vi "PH_Beckhoff.set i Attr and open Services.vi"(0 "i ref in":refnum<vi>, 2 "data in":string, 5 "error in":errorcluster) -> (14 "i ref out":refnum<vi>, 16 "i Attr":T1={"GUI Refs"={"ADS Error"=refnum, "Values"=refnum, "configured?"=refnum, "Connection"=refnum, "IP"=refnum, "Prdc Int [ms]"=refnum}, "operation?"=FALSE, "Default Prdc Interval"=0, "Connection"={"DLL?"=FALSE, "Port?"=FALSE, "Client?"=FALSE, "Ping?"=FALSE, "unsuccessful Pings"=0}, "AMS Net ID"={"DLL path"=path "", "AMS Net ID"={"1st # of IP"=0, "2nd # of IP"=0, "3rd # of IP"=0, "4th # of IP"=0, "In Port"=0, "Out Port"=0}}, "Klemmencluster: # of"={"Offset due to Sonderklemms"=0, "analog Inputs"=0, "analog Outputs"=0, "digital Input Bits"=0, "digital Output Bits"=0}, "Values"={"Sonderklemmen Inputs"=[], "Analog Inputs"=[], "Analog Outputs"=[], "Digital Inputs"=[], "Digital Outputs"=[]}, "IP"="", "Description"="", "configured?"=FALSE, "Change Manager"={"Detemination wanted?"=FALSE, "Values changed at"={"Sonderklemmen Inputs"=[], "Analog Inputs"=[], "Analog Outputs"=[], "Digital Inputs"=[], "Digital Outputs"=[]}}, "Difference to handle an analog input as change"=1}, 19 "error out":errorcluster)   [LabVIEW 2014, in "PH_Beckhoff.lvlib"]
doc: "This VI opens all DIM services."
uses:
  PH_Beckhoff.lvlib
  PH_Beckhoff.i attribute.ctl
  PH_Beckhoff.GUI Refs.ctl
  PH_Beckhoff.Values.ctl
  PH_Beckhoff.Sonderklemmen Inputs.ctl
  PH_Beckhoff.Analog Inputs.ctl
  PH_Beckhoff.Scaling Type.ctl
  PH_Beckhoff.Analog Outputs.ctl
  PH_Beckhoff.Digital Inputs.ctl
  PH_Beckhoff.Digital Outputs.ctl
  PH_Beckhoff.Connectivity.ctl
  non_GPL/instr.lib/Beckhoff/Helpers/Beckhoff Access.ctl
  non_GPL/instr.lib/Beckhoff/Helpers/Klemmendeclarer.ctl
  PH_Beckhoff.constructor Data in.ctl
  lib.lib/DimLVEvent/LVDimInterface/LVDimInterface.lvlib
  non_GPL/instr.lib/Beckhoff/Beckhoff - Driver np.lvlib
  CSCore/CSSystem/CSSystemLib/CSSystemLib.lvlib
  CSCore/BaseProcess/BaseProcess.lvlib
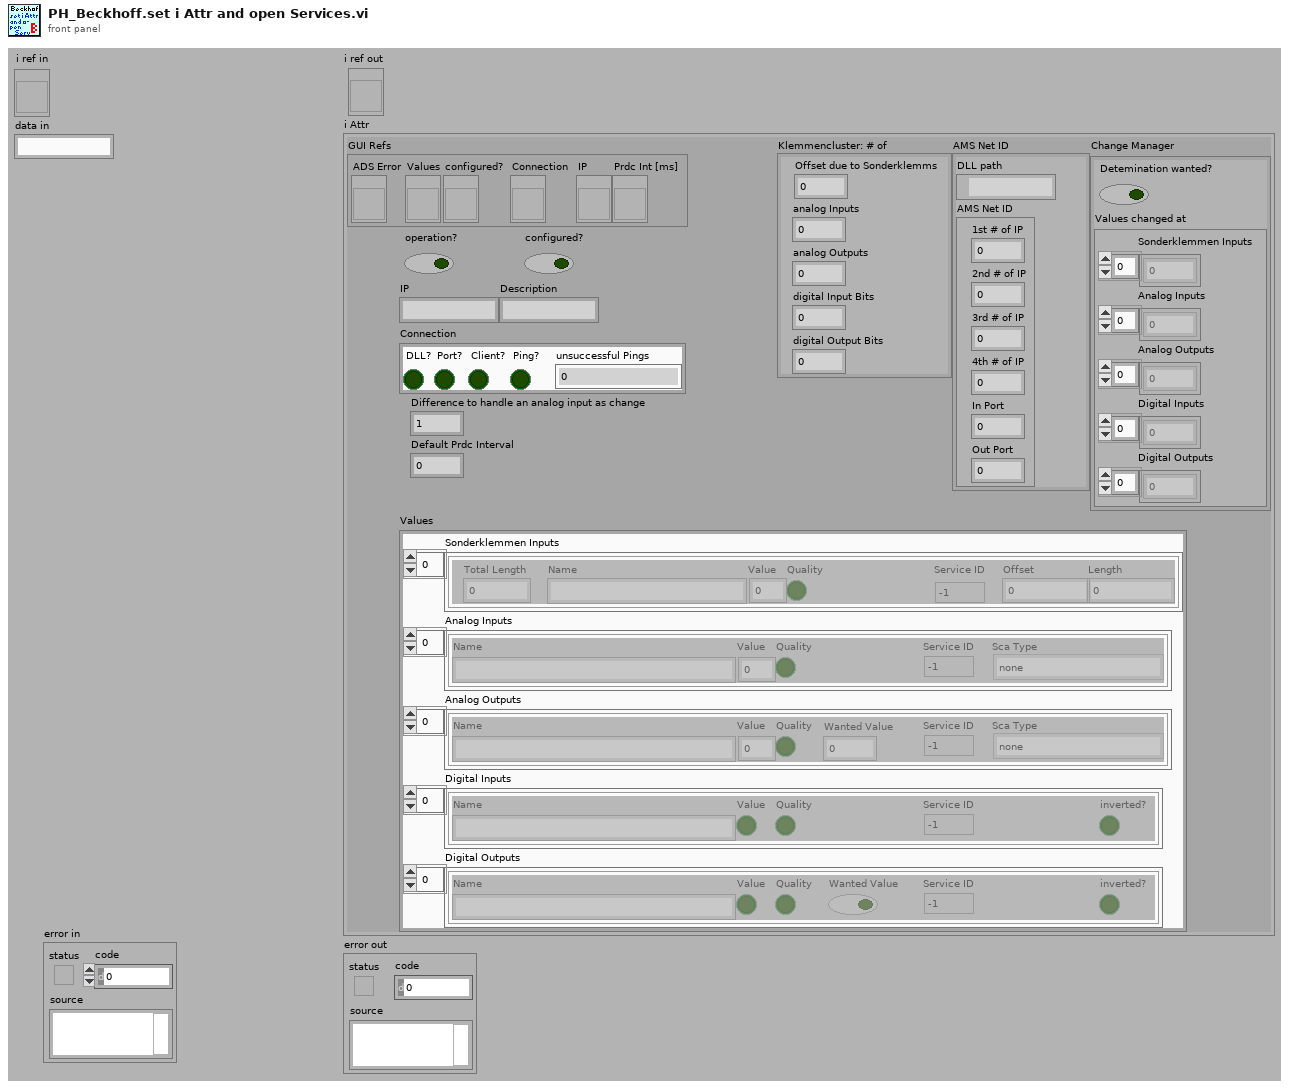
[diagram p1: front panel]
types:
  T1 = typedef "PH_Beckhoff.lvlib/PH_Beckhoff.i attribute.ctl" = cluster{"GUI Refs":T2, "operation?":bool, "Default Prdc Interval":i32, "Connection":T3, "AMS Net ID":T4, "Klemmencluster: # of":T5, "Values":T6, "IP":string, "Description":string, "configured?":bool, "Change Manager":cluster{"Detemination wanted?":bool, "Values changed at":cluster{"Sonderklemmen Inputs":i32[], "Analog Inputs":i32[], "Analog Outputs":i32[], "Digital Inputs":i32[], "Digital Outputs":i32[]}}, "Difference to handle an analog input as change":u32}
  T2 = typedef "PH_Beckhoff.lvlib/PH_Beckhoff.GUI Refs.ctl" = cluster{"ADS Error":refnum<vi>, "Values":refnum<vi>, "configured?":refnum<vi>, "Connection":refnum<vi>, "IP":refnum<vi>, "Prdc Int [ms]":refnum<vi>}
  T3 = typedef "PH_Beckhoff.lvlib/PH_Beckhoff.Connectivity.ctl" = cluster{"DLL?":bool, "Port?":bool, "Client?":bool, "Ping?":bool, "unsuccessful Pings":u32}
  T4 = typedef "Beckhoff - Driver np.lvlib/Beckhoff Access.ctl" = cluster{"DLL path":path, "AMS Net ID":cluster{"1st # of IP":u8, "2nd # of IP":u8, "3rd # of IP":u8, "4th # of IP":u8, "In Port":u8, "Out Port":u8}}
  T5 = typedef "Beckhoff - Driver np.lvlib/Klemmendeclarer.ctl" = cluster{"Offset due to Sonderklemms":u32, "analog Inputs":u32, "analog Outputs":u32, "digital Input Bits":u32, "digital Output Bits":u32}
  T6 = typedef "PH_Beckhoff.lvlib/PH_Beckhoff.Values.ctl" = cluster{"Sonderklemmen Inputs":T7, "Analog Inputs":T8, "Analog Outputs":T10, "Digital Inputs":T11, "Digital Outputs":T12}
  T7 = typedef "PH_Beckhoff.lvlib/PH_Beckhoff.Sonderklemmen Inputs.ctl" = cluster{"Total Length":u32, "Name":string, "Value":u64, "Quality":bool, "Service ID":i32, "Offset":u32, "Length":u32}[]
  T8 = typedef "PH_Beckhoff.lvlib/PH_Beckhoff.Analog Inputs.ctl" = cluster{"Name":string, "Value":u32, "Quality":bool, "Service ID":i32, "Sca Type":T9}[]
  T9 = typedef "PH_Beckhoff.lvlib/PH_Beckhoff.Scaling Type.ctl" = enum16{"none", "0 ... 15 Bit -> 0 ... 5", "0 ... 15 Bit -> 0 ... 10", "0 ... 15 Bit -> 0 ... 25", "0 ... 15 Bit -> 4 ... 20", "0 ... 15 Bit -> 0 ... 1", "0 ... 15 Bit -> 0 ... 20000", "0 ... 15 Bit -> 0 ... 24000"}
  T10 = typedef "PH_Beckhoff.lvlib/PH_Beckhoff.Analog Outputs.ctl" = cluster{"Name":string, "Value":u32, "Quality":bool, "Wanted Value":u32, "Service ID":i32, "Sca Type":T9}[]
  T11 = typedef "PH_Beckhoff.lvlib/PH_Beckhoff.Digital Inputs.ctl" = cluster{"Name":string, "Value":bool, "Quality":bool, "Service ID":i32, "inverted?":bool}[]
  T12 = typedef "PH_Beckhoff.lvlib/PH_Beckhoff.Digital Outputs.ctl" = cluster{"Name":string, "Value":bool, "Quality":bool, "Wanted Value":bool, "Service ID":i32, "inverted?":bool}[]
  T13 = typedef "PH_Beckhoff.lvlib/PH_Beckhoff.constructor Data in.ctl" = cluster{"Default Values":T6, "Description":string, "Hardware configured?":bool, "Activate Change Manager?":bool, "Difference to handle an analog input as change":u32}
  T14 = cluster{"Total Length":u32, "Name":string, "Value":u64, "Quality":bool, "Service ID":i32, "Offset":u32, "Length":u32}
  T15 = cluster{"Name":string, "Value":bool, "Quality":bool, "Wanted Value":bool, "Service ID":i32, "inverted?":bool}
  T16 = cluster{"Name":string, "Value":bool, "Quality":bool, "Service ID":i32, "inverted?":bool}
  T17 = cluster{"Name":string, "Value":u32, "Quality":bool, "Wanted Value":u32, "Service ID":i32, "Sca Type":T9}
  T18 = cluster{"Name":string, "Value":u32, "Quality":bool, "Service ID":i32, "Sca Type":T9}
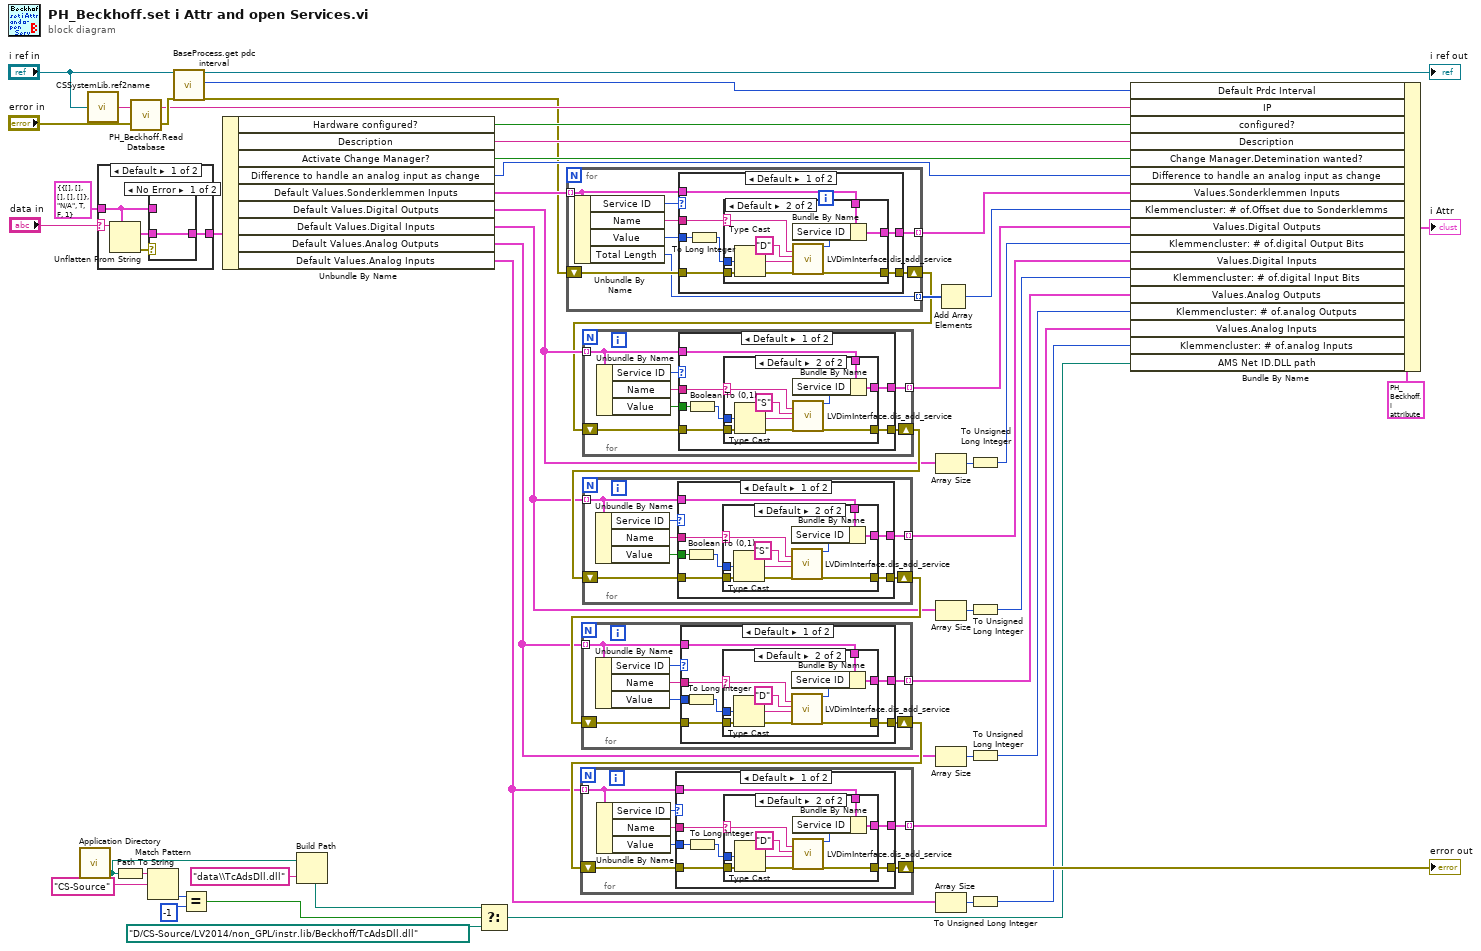
[diagram p0: block diagram]
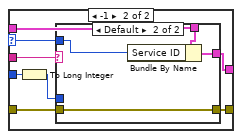
[diagram p5: hidden frame]
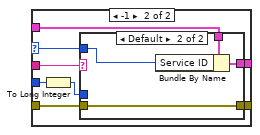
[diagram p8: hidden frame]
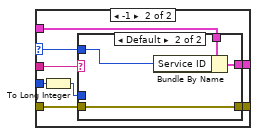
[diagram p11: hidden frame]
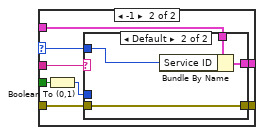
[diagram p14: hidden frame]
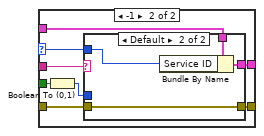
[diagram p17: hidden frame]
diagram:
  n1 = call <vilib>:"Application Directory.vi"() -> ("Application Directory"=w37:path)
  n2 = call "CSSystemLib.ref2name.vi"("obj refnum"="i ref in") -> ("name"=w1:string)
  n3 = case shown="Default" "data in" {
    selector: "data in" -> [w57 _]
    tunnel: T13 {"Default Values"={"Sonderklemmen Inputs"=[], "Analog Inputs"=[], "Analog Outputs"=[], "Digital Inputs"=[], "Digital Outputs"=[]}, "Description"="N/A", "Hardware configured?"=TRUE, "Activate Change Manager?"=FALSE, "Difference to handle an analog input as change"=1} ("data in cluster") -> [w53 w60]
    tunnel: [w54 w60] -> w31
    frame Default {
      n4 = Unflatten From String(type=w53, binary string=w57) -> (value=w55:T13, error out=w56:errorcluster)  [unwired: 3 in, 1 out]
      n5 = case shown="No Error" w56 {
        tunnel: w55 -> [w58 _]
        tunnel: [w58 w59] -> w54
        tunnel: w53 -> [_ w59]
        frame No Error {
        }
        frame Error {
        }
      }
    }
    frame "", "N/A" {
    }
  }
  n6 = Path To String(path=w37) -> (string=w32:string)
  n7 = call "PH_Beckhoff.Read Database.vi"("error in (no error)"="error in", "DB Entry to read"=w1) -> ("error out"=w10:errorcluster, "IP"=w7:string)
  n8 = Match Pattern(string=w32, regular expression="CS-Source") -> (offset past match=w34:i32)  [unwired: 1 in, 3 out]
  n9 = call "BaseProcess.get pdc interval.vi"("i ref in"="i ref in", "error in (no error)"=w10) -> ("i ref out"=→"i ref out":refnum<vi>, "PeriodicInterval"=w9:i32, "error out"=w4:errorcluster)  [unwired: 15 in]
  n10 = Equal?(x=w34, y=-1) -> (x = y?=w36:bool)
  n11 = Unbundle By Name(w31) -> ("Hardware configured?"=w8:bool, "Description"=w14:string, "Activate Change Manager?"=w13:bool, "Difference to handle an analog input as change"=w6:u32, "Default Values.Sonderklemmen Inputs"=w28:T7, "Default Values.Digital Outputs"=w27:T12, "Default Values.Digital Inputs"=w26:T11, "Default Values.Analog Outputs"=w25:T10, "Default Values.Analog Inputs"=w11:T8)
  n12 = Build Path(base path=w37, name or relative path="data\\TcAdsDll.dll") -> (appended path=w39:path)
  n13 = Select(t=w39, s=w36, f=path "D:/CS-Source/LV2014/non_GPL/instr.lib/Beckhoff/TcAdsDll.dll") -> (s? t:f=w15:path)
  n14 = for {
    shift-right: [w67] -> w21
    shift-left: w4 -> [w68]
    tunnel: [w66] -> w23 mode=indexing
    tunnel: w28 -> [w65] mode=indexing
    tunnel: [w62] -> w42 mode=indexing
    n15 = Unbundle By Name(w65) -> ("Service ID"=w61:i32, "Name"=w64:string, "Value"=w63:u64, "Total Length"=w62:u32)
    n16 = case shown="Default" w61 {
      selector: w61 -> [_ w87]
      tunnel: w68 -> [w75 w94]
      tunnel: [w74 w93] -> w67
      tunnel: [w73 w92] -> w66
      tunnel: w65 -> [w72 w91]
      tunnel: w64 -> [w71 w90]
      tunnel: w63 -> [w70 w89]
      frame Default {
        n17 = To Long Integer(number=w70) -> (32bit integer=w69:i32)
        n18 = case shown="Default" w71 {
          selector: w71 -> [_ w78]
          tunnel: w75 -> [w76 w84]
          tunnel: [w76 w83] -> w74
          tunnel: [w77 w81] -> w73
          tunnel: w72 -> [w77 w80]
          tunnel: w69 -> [_ w79]
          frame "", "N/A" {
          }
          frame Default {
            n19 = Type Cast(x=w79) -> (*(type *) &x=w86:string)  [unwired: 1 in]
            n20 = call "LVDimInterface.dis_add_service.vi"("serviceName"=w78, "typeDescriptor"="D", "data"=w86, "error in (no error)"=w84) -> ("my_serviceID"=w82:i32, "error out"=w83:errorcluster)  [unwired: 14 in]
            n21 = Bundle By Name(cluster=w80, "Service ID"=w82) -> (w81:T14)
          }
        }
      }
      frame -1 {
        n22 = To Long Integer(number=w89) -> (32bit integer=w88:i32)
        n23 = case shown="Default" w90 {
          tunnel: w94 -> [w95 w98]
          tunnel: [w95 w98] -> w93
          tunnel: [w96 w100] -> w92
          tunnel: w91 -> [w96 w99]
          tunnel: w88 -> [_ _]
          tunnel: w87 -> [_ w97]
          frame "", "N/A" {
          }
          frame Default {
            n24 = Bundle By Name(cluster=w99, "Service ID"=w97) -> (w100:T14)
          }
        }
      }
    }
  }
  n25 = for {
    shift-right: [w106] -> w45
    shift-left: w21 -> [w107]
    tunnel: [w105] -> w52 mode=indexing
    tunnel: w27 -> [w104] mode=indexing
    n26 = Unbundle By Name(w104) -> ("Service ID"=w101:i32, "Name"=w103:string, "Value"=w102:bool)
    n27 = case shown="Default" w101 {
      selector: w101 -> [_ w126]
      tunnel: w107 -> [w114 w133]
      tunnel: [w113 w132] -> w106
      tunnel: [w112 w131] -> w105
      tunnel: w104 -> [w111 w130]
      tunnel: w103 -> [w110 w129]
      tunnel: w102 -> [w109 w128]
      frame Default {
        n28 = Boolean To (0,1)(Boolean=w109) -> (0, 1=w108:i16)
        n29 = case shown="Default" w110 {
          selector: w110 -> [_ w117]
          tunnel: w114 -> [w115 w123]
          tunnel: [w115 w122] -> w113
          tunnel: [w116 w120] -> w112
          tunnel: w111 -> [w116 w119]
          tunnel: w108 -> [_ w118]
          frame "", "N/A" {
          }
          frame Default {
            n30 = Type Cast(x=w118) -> (*(type *) &x=w125:string)  [unwired: 1 in]
            n31 = call "LVDimInterface.dis_add_service.vi"("serviceName"=w117, "typeDescriptor"="S", "data"=w125, "error in (no error)"=w123) -> ("my_serviceID"=w121:i32, "error out"=w122:errorcluster)  [unwired: 14 in]
            n32 = Bundle By Name(cluster=w119, "Service ID"=w121) -> (w120:T15)
          }
        }
      }
      frame -1 {
        n33 = Boolean To (0,1)(Boolean=w128) -> (0, 1=w127:i16)
        n34 = case shown="Default" w129 {
          tunnel: w133 -> [w134 w137]
          tunnel: [w134 w137] -> w132
          tunnel: [w135 w139] -> w131
          tunnel: w130 -> [w135 w138]
          tunnel: w127 -> [_ _]
          tunnel: w126 -> [_ w136]
          frame "", "N/A" {
          }
          frame Default {
            n35 = Bundle By Name(cluster=w138, "Service ID"=w136) -> (w139:T15)
          }
        }
      }
    }
  }
  n36 = for {
    shift-right: [w145] -> w43
    shift-left: w45 -> [w146]
    tunnel: [w144] -> w51 mode=indexing
    tunnel: w26 -> [w141] mode=indexing
    n37 = Unbundle By Name(w141) -> ("Service ID"=w140:i32, "Name"=w143:string, "Value"=w142:bool)
    n38 = case shown="Default" w140 {
      selector: w140 -> [_ w165]
      tunnel: w146 -> [w153 w172]
      tunnel: [w152 w171] -> w145
      tunnel: [w151 w170] -> w144
      tunnel: w143 -> [w150 w169]
      tunnel: w142 -> [w149 w168]
      tunnel: w141 -> [w147 w166]
      frame Default {
        n39 = Boolean To (0,1)(Boolean=w149) -> (0, 1=w148:i16)
        n40 = case shown="Default" w150 {
          selector: w150 -> [_ w156]
          tunnel: w153 -> [w154 w162]
          tunnel: [w154 w161] -> w152
          tunnel: [w155 w159] -> w151
          tunnel: w147 -> [w155 w158]
          tunnel: w148 -> [_ w157]
          frame "", "N/A" {
          }
          frame Default {
            n41 = Type Cast(x=w157) -> (*(type *) &x=w164:string)  [unwired: 1 in]
            n42 = call "LVDimInterface.dis_add_service.vi"("serviceName"=w156, "typeDescriptor"="S", "data"=w164, "error in (no error)"=w162) -> ("my_serviceID"=w160:i32, "error out"=w161:errorcluster)  [unwired: 14 in]
            n43 = Bundle By Name(cluster=w158, "Service ID"=w160) -> (w159:T16)
          }
        }
      }
      frame -1 {
        n44 = Boolean To (0,1)(Boolean=w168) -> (0, 1=w167:i16)
        n45 = case shown="Default" w169 {
          tunnel: w172 -> [w173 w176]
          tunnel: [w173 w176] -> w171
          tunnel: [w174 w178] -> w170
          tunnel: w166 -> [w174 w177]
          tunnel: w167 -> [_ _]
          tunnel: w165 -> [_ w175]
          frame "", "N/A" {
          }
          frame Default {
            n46 = Bundle By Name(cluster=w177, "Service ID"=w175) -> (w178:T16)
          }
        }
      }
    }
  }
  n47 = for {
    shift-right: [w184] -> w44
    shift-left: w43 -> [w185]
    tunnel: [w183] -> w50 mode=indexing
    tunnel: w25 -> [w182] mode=indexing
    n48 = Unbundle By Name(w182) -> ("Service ID"=w179:i32, "Name"=w181:string, "Value"=w180:u32)
    n49 = case shown="Default" w179 {
      selector: w179 -> [_ w204]
      tunnel: w185 -> [w192 w211]
      tunnel: [w191 w210] -> w184
      tunnel: [w190 w209] -> w183
      tunnel: w182 -> [w189 w208]
      tunnel: w181 -> [w188 w207]
      tunnel: w180 -> [w187 w206]
      frame Default {
        n50 = To Long Integer(number=w187) -> (32bit integer=w186:i32)
        n51 = case shown="Default" w188 {
          selector: w188 -> [_ w195]
          tunnel: w192 -> [w193 w201]
          tunnel: [w193 w200] -> w191
          tunnel: [w194 w198] -> w190
          tunnel: w189 -> [w194 w197]
          tunnel: w186 -> [_ w196]
          frame "", "N/A" {
          }
          frame Default {
            n52 = Type Cast(x=w196) -> (*(type *) &x=w203:string)  [unwired: 1 in]
            n53 = call "LVDimInterface.dis_add_service.vi"("serviceName"=w195, "typeDescriptor"="D", "data"=w203, "error in (no error)"=w201) -> ("my_serviceID"=w199:i32, "error out"=w200:errorcluster)  [unwired: 14 in]
            n54 = Bundle By Name(cluster=w197, "Service ID"=w199) -> (w198:T17)
          }
        }
      }
      frame -1 {
        n55 = To Long Integer(number=w206) -> (32bit integer=w205:i32)
        n56 = case shown="Default" w207 {
          tunnel: w211 -> [w212 w215]
          tunnel: [w212 w215] -> w210
          tunnel: [w213 w217] -> w209
          tunnel: w208 -> [w213 w216]
          tunnel: w205 -> [_ _]
          tunnel: w204 -> [_ w214]
          frame "", "N/A" {
          }
          frame Default {
            n57 = Bundle By Name(cluster=w216, "Service ID"=w214) -> (w217:T17)
          }
        }
      }
    }
  }
  n58 = for {
    shift-right: [w223] -> w20
    shift-left: w44 -> [w224]
    tunnel: [w222] -> w12 mode=indexing
    tunnel: w11 -> [w221] mode=indexing
    n59 = Unbundle By Name(w221) -> ("Service ID"=w218:i32, "Name"=w220:string, "Value"=w219:u32)
    n60 = case shown="Default" w218 {
      selector: w218 -> [_ w243]
      tunnel: w224 -> [w231 w250]
      tunnel: [w230 w249] -> w223
      tunnel: [w229 w248] -> w222
      tunnel: w221 -> [w228 w247]
      tunnel: w220 -> [w227 w246]
      tunnel: w219 -> [w226 w245]
      frame Default {
        n61 = To Long Integer(number=w226) -> (32bit integer=w225:i32)
        n62 = case shown="Default" w227 {
          selector: w227 -> [_ w234]
          tunnel: w231 -> [w232 w240]
          tunnel: [w232 w239] -> w230
          tunnel: [w233 w237] -> w229
          tunnel: w228 -> [w233 w236]
          tunnel: w225 -> [_ w235]
          frame "", "N/A" {
          }
          frame Default {
            n63 = Type Cast(x=w235) -> (*(type *) &x=w242:string)  [unwired: 1 in]
            n64 = call "LVDimInterface.dis_add_service.vi"("serviceName"=w234, "typeDescriptor"="D", "data"=w242, "error in (no error)"=w240) -> ("my_serviceID"=w238:i32, "error out"=w239:errorcluster)  [unwired: 14 in]
            n65 = Bundle By Name(cluster=w236, "Service ID"=w238) -> (w237:T18)
          }
        }
      }
      frame -1 {
        n66 = To Long Integer(number=w245) -> (32bit integer=w244:i32)
        n67 = case shown="Default" w246 {
          tunnel: w250 -> [w251 w254]
          tunnel: [w251 w254] -> w249
          tunnel: [w252 w256] -> w248
          tunnel: w247 -> [w252 w255]
          tunnel: w244 -> [_ _]
          tunnel: w243 -> [_ w253]
          frame "", "N/A" {
          }
          frame Default {
            n68 = Bundle By Name(cluster=w255, "Service ID"=w253) -> (w256:T18)
          }
        }
      }
    }
  }
  "error out" <- w20
  n69 = Array Size(array=w27) -> (size(s)=w49:i32)
  n70 = Array Size(array=w26) -> (size(s)=w46:i32)
  n71 = Array Size(array=w25) -> (size(s)=w47:i32)
  n72 = Array Size(array=w11) -> (size(s)=w48:i32)
  n73 = Add Array Elements(numeric array=w42) -> (sum=w22:u32)
  n74 = To Unsigned Long Integer(number=w49) -> (unsigned 32bit integer=w19:u32)
  n75 = To Unsigned Long Integer(number=w46) -> (unsigned 32bit integer=w18:u32)
  n76 = To Unsigned Long Integer(number=w47) -> (unsigned 32bit integer=w17:u32)
  n77 = To Unsigned Long Integer(number=w48) -> (unsigned 32bit integer=w16:u32)
  n78 = Bundle By Name(cluster=T1 {"GUI Refs"={"ADS Error"=refnum, "Values"=refnum, "configured?"=refnum, "Connection"=refnum, "IP"=refnum, "Prdc Int [ms]"=refnum}, "operation?"=FALSE, "Default Prdc Interval"=0, "Connection"={"DLL?"=FALSE, "Port?"=FALSE, "Client?"=FALSE, "Ping?"=FALSE, "unsuccessful Pings"=0}, "AMS Net ID"={"DLL path"=path "", "AMS Net ID"={"1st # of IP"=0, "2nd # of IP"=0, "3rd # of IP"=0, "4th # of IP"=0, "In Port"=0, "Out Port"=0}}, "Klemmencluster: # of"={"Offset due to Sonderklemms"=0, "analog Inputs"=0, "analog Outputs"=0, "digital Input Bits"=0, "digital Output Bits"=0}, "Values"={"Sonderklemmen Inputs"=[], "Analog Inputs"=[], "Analog Outputs"=[], "Digital Inputs"=[], "Digital Outputs"=[]}, "IP"="", "Description"="", "configured?"=FALSE, "Change Manager"={"Detemination wanted?"=FALSE, "Values changed at"={"Sonderklemmen Inputs"=[], "Analog Inputs"=[], "Analog Outputs"=[], "Digital Inputs"=[], "Digital Outputs"=[]}}, "Difference to handle an analog input as change"=1} ("i Attr 2"), "Default Prdc Interval"=w9, "IP"=w7, "configured?"=w8, "Description"=w14, "Change Manager.Detemination wanted?"=w13, "Difference to handle an analog input as change"=w6, "Values.Sonderklemmen Inputs"=w23, "Klemmencluster: # of.Offset due to Sonderklemms"=w22, "Values.Digital Outputs"=w52, "Klemmencluster: # of.digital Output Bits"=w19, "Values.Digital Inputs"=w51, "Klemmencluster: # of.digital Input Bits"=w18, "Values.Analog Outputs"=w50, "Klemmencluster: # of.analog Outputs"=w17, "Values.Analog Inputs"=w12, "Klemmencluster: # of.analog Inputs"=w16, "AMS Net ID.DLL path"=w15) -> (→"i Attr":T1)
